vi "fpga_check_threshold.vi"(7 "threshold":T3, 10 "feedback":T2, 11 "input":T1) -> (3 "inrange?":bool)   [LabVIEW 2021]
doc: "Check if the data is inrage or not."
uses:
  fpga_dtype_threshold.ctl
  fpga_dtype_sgl_8ch.ctl
  fpga_dtype_sgl_fb.ctl
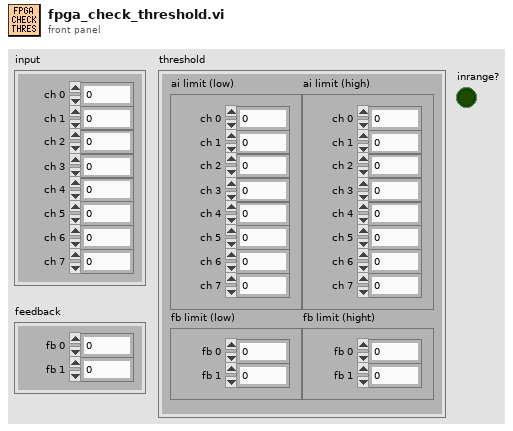
[diagram p1: front panel]
types:
  T1 = typedef "fpga_dtype_sgl_8ch.ctl" = cluster{"ch 0":sgl, "ch 1":sgl, "ch 2":sgl, "ch 3":sgl, "ch 4":sgl, "ch 5":sgl, "ch 6":sgl, "ch 7":sgl}
  T2 = typedef "fpga_dtype_sgl_fb.ctl" = cluster{"fb 0":sgl, "fb 1":sgl}
  T3 = typedef "fpga_dtype_threshold.ctl" = cluster{"ai limit (high)":T1, "fb limit (hight)":T2, "ai limit (low)":T1, "fb limit (low)":T2}
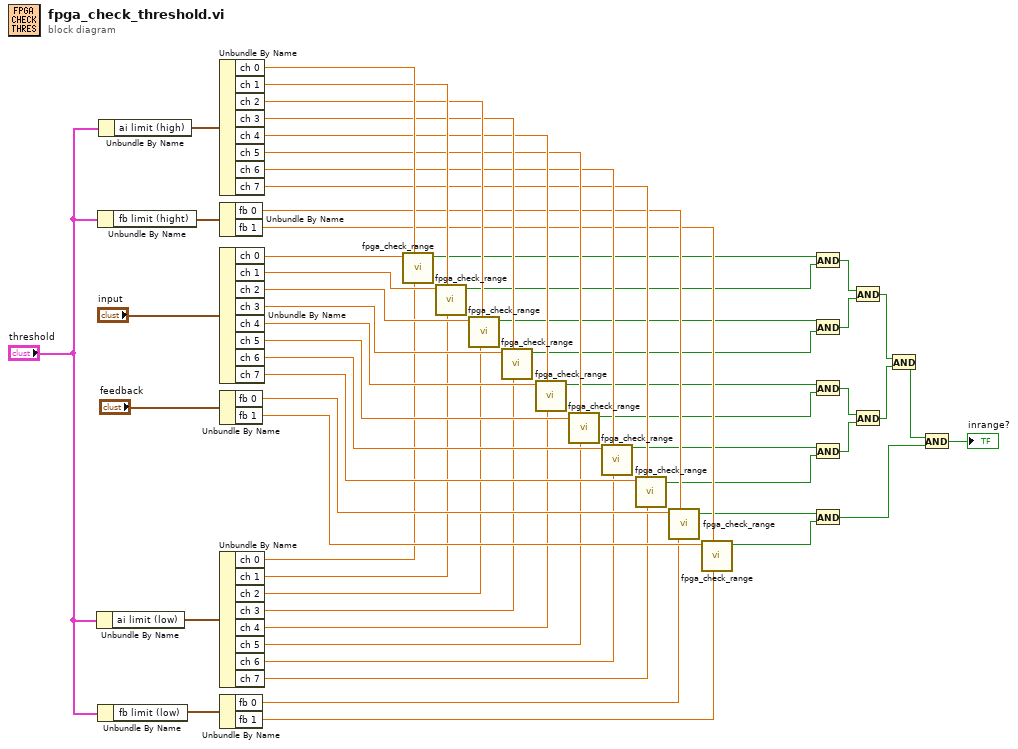
[diagram p0: block diagram]
diagram:
  n1 = Unbundle By Name("threshold") -> ("ai limit (low)"=w52:T1)
  n2 = Unbundle By Name("threshold") -> ("fb limit (hight)"=w51:T2)
  n3 = Unbundle By Name("threshold") -> ("fb limit (low)"=w53:T2)
  n4 = Unbundle By Name("threshold") -> ("ai limit (high)"=w54:T1)
  n5 = Unbundle By Name(w54) -> ("ch 0"=w29:sgl, "ch 1"=w28:sgl, "ch 2"=w27:sgl, "ch 3"=w26:sgl, "ch 4"=w25:sgl, "ch 5"=w24:sgl, "ch 6"=w23:sgl, "ch 7"=w22:sgl)
  n6 = Unbundle By Name(w51) -> ("fb 0"=w21:sgl, "fb 1"=w20:sgl)
  n7 = Unbundle By Name("input") -> ("ch 0"=w49:sgl, "ch 1"=w48:sgl, "ch 2"=w47:sgl, "ch 3"=w46:sgl, "ch 4"=w45:sgl, "ch 5"=w44:sgl, "ch 6"=w43:sgl, "ch 7"=w42:sgl)
  n8 = Unbundle By Name("feedback") -> ("fb 0"=w41:sgl, "fb 1"=w40:sgl)
  n9 = Unbundle By Name(w52) -> ("ch 0"=w39:sgl, "ch 1"=w38:sgl, "ch 2"=w37:sgl, "ch 3"=w36:sgl, "ch 4"=w35:sgl, "ch 5"=w34:sgl, "ch 6"=w33:sgl, "ch 7"=w32:sgl)
  n10 = Unbundle By Name(w53) -> ("fb 0"=w31:sgl, "fb 1"=w30:sgl)
  n11 = call "fpga_check_range.vi"("limit (low)"=w39, "limit (high)"=w29, "value"=w49) -> ("inrange?"=w19:bool)  [unwired: 8 in]
  n12 = call "fpga_check_range.vi"("limit (low)"=w38, "limit (high)"=w28, "value"=w48) -> ("inrange?"=w18:bool)  [unwired: 8 in]
  n13 = call "fpga_check_range.vi"("limit (low)"=w37, "limit (high)"=w27, "value"=w47) -> ("inrange?"=w17:bool)  [unwired: 8 in]
  n14 = call "fpga_check_range.vi"("limit (low)"=w36, "limit (high)"=w26, "value"=w46) -> ("inrange?"=w16:bool)  [unwired: 8 in]
  n15 = call "fpga_check_range.vi"("limit (low)"=w35, "limit (high)"=w25, "value"=w45) -> ("inrange?"=w15:bool)  [unwired: 8 in]
  n16 = call "fpga_check_range.vi"("limit (low)"=w34, "limit (high)"=w24, "value"=w44) -> ("inrange?"=w14:bool)  [unwired: 8 in]
  n17 = call "fpga_check_range.vi"("limit (low)"=w33, "limit (high)"=w23, "value"=w43) -> ("inrange?"=w13:bool)  [unwired: 8 in]
  n18 = call "fpga_check_range.vi"("limit (low)"=w32, "limit (high)"=w22, "value"=w42) -> ("inrange?"=w12:bool)  [unwired: 8 in]
  n19 = call "fpga_check_range.vi"("limit (low)"=w31, "limit (high)"=w21, "value"=w41) -> ("inrange?"=w11:bool)  [unwired: 8 in]
  n20 = call "fpga_check_range.vi"("limit (low)"=w30, "limit (high)"=w20, "value"=w40) -> ("inrange?"=w10:bool)  [unwired: 8 in]
  n21 = And(x=w19, y=w18) -> (x .and. y?=w9:bool)
  n22 = And(x=w17, y=w16) -> (x .and. y?=w8:bool)
  n23 = And(x=w15, y=w14) -> (x .and. y?=w7:bool)
  n24 = And(x=w13, y=w12) -> (x .and. y?=w6:bool)
  n25 = And(x=w11, y=w10) -> (x .and. y?=w1:bool)
  n26 = And(x=w9, y=w8) -> (x .and. y?=w5:bool)
  n27 = And(x=w7, y=w6) -> (x .and. y?=w4:bool)
  n28 = And(x=w5, y=w4) -> (x .and. y?=w3:bool)
  n29 = And(x=w3, y=w1) -> (x .and. y?=→"inrange?":bool)
